vi "z shm clone.vi"(8 "error in (no error)":errorcluster, 10 "this_":cluster{}, 11 "out":cluster{}) -> (0 "error out":errorcluster, 3 "out out":cluster{})   [LabVIEW 2021, in "zenohc.lvlib"]
doc: "void z_shm_clone(struct z_owned_shm_t *out,\n const struct z_loaned_shm_t *this_);"
uses:
  zenohc.lvlib
  zenohc.dll
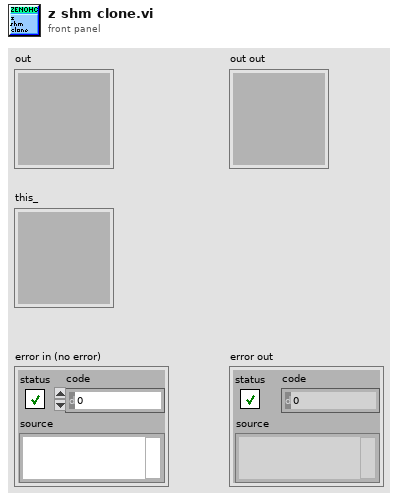
[diagram p1: front panel]
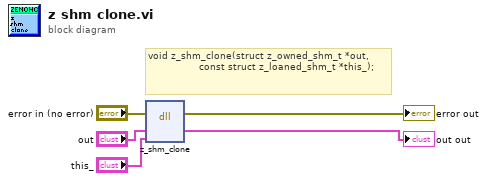
[diagram p0: block diagram]
diagram:
  # "void z_shm_clone(struct z_owned_shm_t *out,\n                 const struct z_loaned_shm_t *this_);"
  n1 = dll-call lib="D:/dev/zenoh_labview/zenohc/zenohc.*" fn="z_shm_clone"(error in="error in (no error)", "out"="out", "this_"="this_") -> (error out=→"error out":errorcluster, "out"=→"out out":cluster{})  [unwired: 4 in, 1 out]
